vi "driveCode.vi"   [LabVIEW 2016]
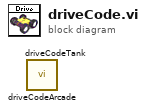
[diagram p0: block diagram]
diagram:
  n1 = call "driveCodeArcade.vi"() -> ()  [unwired: 8 in, 4 out]
  n2 = call "driveCodeTank.vi"() -> ()  [unwired: 8 in, 4 out]
